vi "Load_HistoryUpdate.vi"(0 "Limit to 30":bool, 2 "History ref":refnum<vi>, 3 "New Path":string) -> ()   [LabVIEW 2013]
doc: "This VI adds the \"New Path\" to the history, provided it is not already an element. Pre-existing duplicates are not removed."
panel:
  out "History Out":string[](array[string])
  out "History in":string[](array[string])
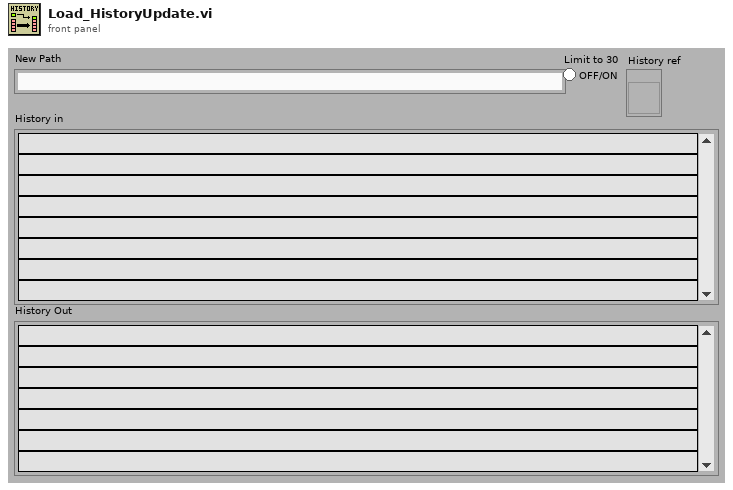
[diagram p1: front panel]
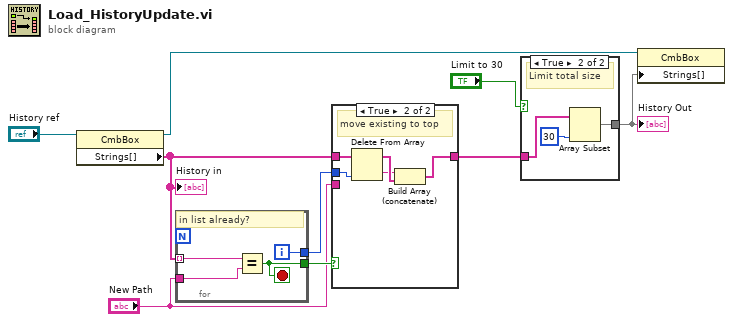
[diagram p0: block diagram]
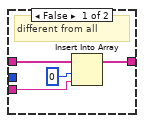
[diagram p3: hidden frame]
diagram:
  n1 = property class="CmbBox"(reference="History ref") -> (reference out=w7:refnum<vi>, "Strings[]"=w8:string[])  [unwired: 1 in, 1 out]
  "History in" <- w8
  n2 = for {
    tunnel: w8 -> [w13] mode=indexing
    tunnel: "New Path" -> [w12]
    tunnel: [w11] -> w6
    tunnel: [w10] -> w5
    i -> [w11]
    stop <- w10 stop-if-true
    # "in list already?"
    n3 = Equal?(x=w13, y=w12) -> (x = y?=w10:bool)
  }
  n4 = case shown="True" w5 {
    tunnel: w8 -> [w16 w22]
    tunnel: [w15 w20] -> w3
    tunnel: "New Path" -> [w14 _]
    tunnel: w6 -> [_ w21]
    frame False {
      # "different from all"
      n5 = Insert Into Array(array=w16, index=0, new element=w14) -> (w15:string[])
    }
    frame True {
      # "move existing to top"
      n6 = Delete From Array(array=w22, index=w21) -> (deleted portion=w18:string, array with subset deleted=w19:string[])  [unwired: 1 in]
      n7 = Build Array (concatenate)(w18, w19) -> (w20:string[])
    }
  }
  n8 = case shown="True" "Limit to 30" {
    tunnel: w3 -> [w23 w25]
    tunnel: [w23 w24] -> w2
    frame False {
    }
    frame True {
      # "Limit total size"
      n9 = Array Subset(array=w25, length=30) -> (w24:string[])  [unwired: 1 in]
    }
  }
  "History Out" <- w2
  n10 = property class="CmbBox"(reference=w7, "Strings[]"=w2) -> ()  [unwired: 1 in, 2 out]
